vi "SubpanelTestsForEXE.vi"(0 "EXE Path":path, 5 "Drona Tests PPL":path, 11 "Error In":errorcluster) -> (15 "Error Out":errorcluster)   [LabVIEW 2016]
doc: "Run EXE and Load test VI into EXE to run tests in the application"
uses:
  Drona.lvlib
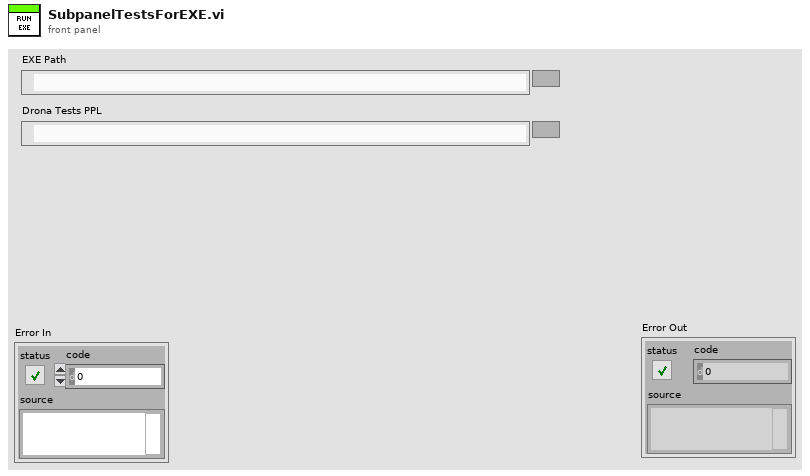
[diagram p1: front panel]
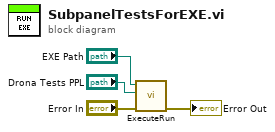
[diagram p0: block diagram]
diagram:
  n1 = call "ExecuteRun.vi"("error in (no error)"="Error In", "Drona Tests PPL"="Drona Tests PPL", "EXE Path"="EXE Path") -> ("error out"=→"Error Out":errorcluster)  [unwired: 8 in]
